vi "Aiming v2.vi"(6 "PID Cluster":T2={"L1 to L4 PID Cluster"={"L1 PID Gains"={"Kp"=0.005, "Kd"=0.5, "Ki"=0.0005}, "L2 PID Gains"={"Kp"=0.01, "Kd"=1.0, "Ki"=0.005}, "L3 PID Gains"={"Kp"=0.05, "Kd"=1.0, "Ki"=0.0005}, "L4 PID Gains"={"Kp"=0.1, "Kd"=0.1, "Ki"=0.0005}}, "Stage PID Cluster"={"Stage Z PID"={"Kp"=0.0005, "Kd"=0.001, "Ki"=0.0}, "Stage Y PID"={"Kp"=0.0003, "Kd"=0.01, "Ki"=0.0}, "Stage X PID"={"Kp"=0.0003, "Kd"=0.01, "Ki"=0.0}}, "OCT Z PID Gains"={"Kp"=0.0003, "Kd"=0.0001, "Ki"=0.01}}, 7 "Robot In":i32, 8 "error in":errorcluster, 9 "Aiming Pt":dbl[](array[numeric])=[0.0, 0.0, 0.0, 0.0], 10 "Prev Posit Cluster":T3={"Prev L1 to L4 Posit"=[0.0, 0.0, 0.0, 0.0], "Prev Stage Posit"=[6.0, 6.0, 6.0], "Prev OCT Z Posit"=0.0}, 11 "FPGA VI Reference In":refnum<k20>) -> (0 "error out":errorcluster, 2 "Last Posit Cluster":T1={"Last L1 to L4 Posit"=[0.0, 0.0, 0.0, 0.0], "Last Stage Posit"=[6.0, 6.0, 6.0], "Last OCT Z Posit"=0.0}, 3 "FPGA VI Reference Out":refnum<k20>)   [LabVIEW 2016]
uses:
  Subsystems/Global Variables.vi
  <vilib>/Platform/TimedLoop/XDataNode/wakeup.ctl
  <vilib>/Platform/TimedLoop/XDataNode/XDNodeRunTimeDep.lvlib
  <vilib>/Platform/TimedLoop/XDataNode/nitl_modes.ctl
  <vilib>/Platform/TimedLoop/XDataNode/timing_clust.ctl
  <vilib>/platform/TimedLoop/XDataNode/XDataNode.xnode
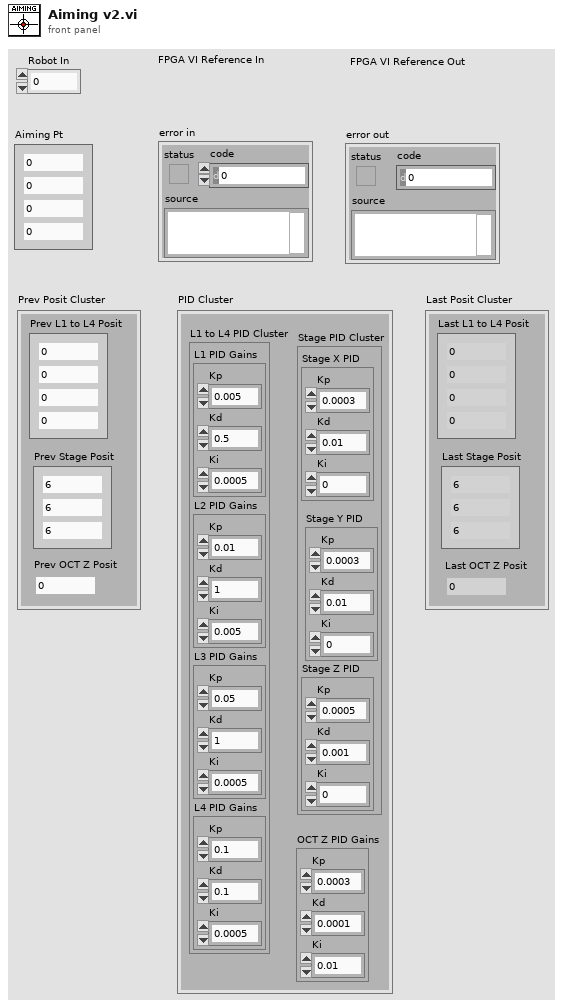
[diagram p1: front panel]
types:
  T1 = cluster{"Last L1 to L4 Posit":dbl[], "Last Stage Posit":dbl[], "Last OCT Z Posit":dbl}
  T2 = cluster{"L1 to L4 PID Cluster":cluster{"L1 PID Gains":cluster{"Kp":dbl, "Kd":dbl, "Ki":dbl}, "L2 PID Gains":cluster{"Kp":dbl, "Kd":dbl, "Ki":dbl}, "L3 PID Gains":cluster{"Kp":dbl, "Kd":dbl, "Ki":dbl}, "L4 PID Gains":cluster{"Kp":dbl, "Kd":dbl, "Ki":dbl}}, "Stage PID Cluster":cluster{"Stage Z PID":cluster{"Kp":dbl, "Kd":dbl, "Ki":dbl}, "Stage Y PID":cluster{"Kp":dbl, "Kd":dbl, "Ki":dbl}, "Stage X PID":cluster{"Kp":dbl, "Kd":dbl, "Ki":dbl}}, "OCT Z PID Gains":cluster{"Kp":dbl, "Kd":dbl, "Ki":dbl}}
  T3 = cluster{"Prev L1 to L4 Posit":dbl[], "Prev Stage Posit":dbl[], "Prev OCT Z Posit":dbl}
  T4 = typedef "XDNodeRunTimeDep.lvlib/timing_clust.ctl" = cluster{"Expected End [f-1]":u64, "Actual End [f-1]":u64, "Finished Late? [f-1]":bool, "Expected End [i-1]":u64, "Actual End [i-1]":u64, "Finished Late? [i-1]":bool, "Expected Start [i]":u64, "Actual Start [i]":u64, "Expected Start [f]":u64, "Actual Start [f]":u64, "Source Name":string, "Structure Name":string, "Period":i64, "Deadline":i64, "Offset":i64, "Start":i64, "Priority":i32, "Timeout":i32, "Mode":T5, "Wakeup Reason":T6, "Error":errorcluster, "Source Type":string, "Secondary Source Type":string, "Global End Time":u64, "Global Start Time":u64, "Frame Duration":u64, "Iteration Duration":u64, "Assigned CPU":i32, "I/O Scan Engine Mode":u32}
  T5 = typedef "XDNodeRunTimeDep.lvlib/nitl_modes.ctl" = enum32{"No Change", "Process missed periods, maintain original phase", "Discard missed periods, maintain original phase", "Process missed periods, ignore original phase", "Discard missed periods, ignore original phase"}
  T6 = typedef "XDNodeRunTimeDep.lvlib/wakeup.ctl" = enum32{"Normal", "Aborted", "Asynchronous wakeup", "Timing source error", "Timed loop error", "Timeout"}
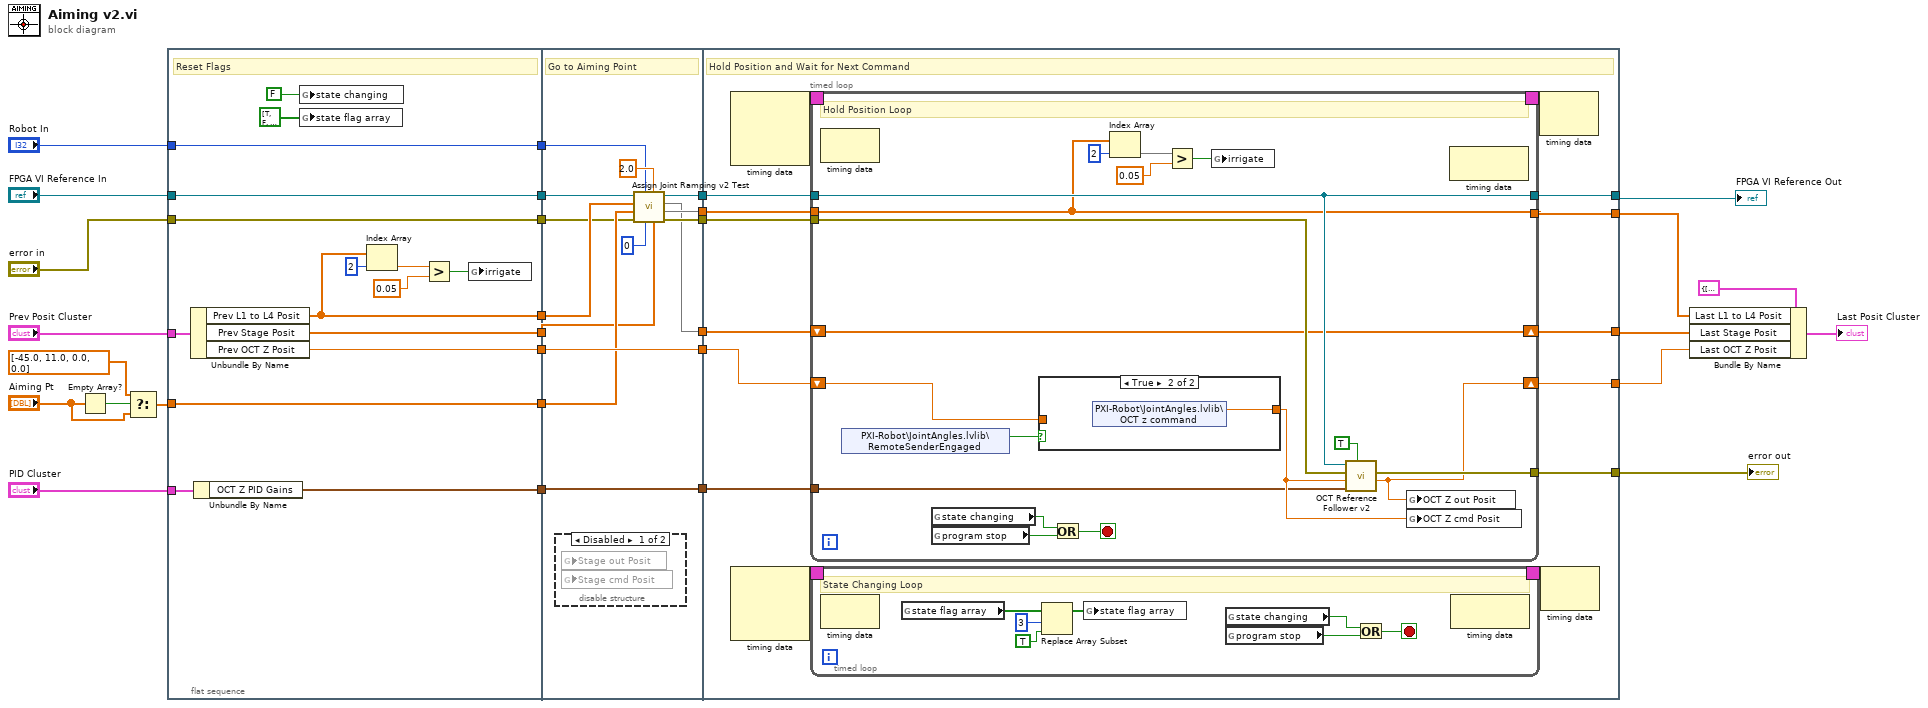
[diagram p0: block diagram]
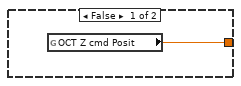
[diagram p3: hidden frame]
diagram:
  n1 = Empty Array?(array="Aiming Pt") -> (empty?=w24:bool)
  n2 = Select(t=dbl[] [-45.0, 11.0, 0.0, 0.0] ("First Trk Pt 2"), s=w24, f="Aiming Pt") -> (s? t:f=w21:dbl[])
  n3 = flat-sequence {
    tunnel: [w44] -> w30
    tunnel: "FPGA VI Reference In" -> [w44]
    tunnel: "error in" -> [w43]
    tunnel: [w43] -> w29
    tunnel: [w31] -> w28
    tunnel: "PID Cluster" -> [w38]
    tunnel: [w39] -> w26
    tunnel: w21 -> [w39]
    tunnel: "Prev Posit Cluster" -> [w42]
    tunnel: [w41] -> w9
    tunnel: [w40] -> w6
    tunnel: [w37] -> w5
    tunnel: "Robot In" -> [w36]
    tunnel: [w36] -> w1
    tunnel: w30 -> [w55]
    tunnel: w29 -> [w52]
    tunnel: w28 -> [w54]
    tunnel: w26 -> [w53]
    tunnel: [w56] -> w25
    tunnel: [w58] -> w20
    tunnel: [w59] -> w17
    tunnel: w9 -> [w48]
    tunnel: [w47] -> w8
    tunnel: [w60] -> w7
    tunnel: w6 -> [w60]
    tunnel: w5 -> [w59]
    tunnel: [w57] -> w4
    tunnel: w1 -> [w50]
    tunnel: [w71] -> w13
    tunnel: w25 -> [w72]
    tunnel: w20 -> [w73]
    tunnel: [w63] -> w18
    tunnel: [w70] -> w19
    tunnel: w17 -> [w69]
    tunnel: [w68] -> w14
    tunnel: [w67] -> w3
    tunnel: w8 -> [w66]
    tunnel: w7 -> [w65]
    tunnel: w4 -> [w64]
    frame #0 {
      # "Reset Flags"
      n4 = Unbundle By Name(w42) -> ("Prev L1 to L4 Posit"=w31:dbl[], "Prev Stage Posit"=w41:dbl[], "Prev OCT Z Posit"=w40:dbl)
      n5 = Unbundle By Name(w38) -> ("OCT Z PID Gains"=w37:cluster{"Kp":dbl, "Kd":dbl, "Ki":dbl})
      n6 = global write "Global Variables.vi" "state changing"(FALSE ("state changing")) -> ()
      n7 = global write "Global Variables.vi" "state flag array"(bool[] [TRUE, FALSE, FALSE, FALSE, FALSE, FALSE, FALSE, FALSE, FALSE] ("state flag array")) -> ()
      n8 = Index Array(array=w31, index=2) -> (element=w34:dbl)
      n9 = Greater?(x=w34, y=0.05) -> (0:w33:bool)
      n10 = global write "Global Variables.vi" "irrigate"(w33) -> ()
    }
    frame #1 {
      # "Go to Aiming Point"
      n11 = disable-structure shown="Disabled" {
        frame Disabled {
          n12 = global read "Global Variables.vi" "Stage out Posit"() -> ()  [unwired: 1 in]
          n13 = global read "Global Variables.vi" "Stage cmd Posit"() -> ()  [unwired: 1 in]
        }
        frame Enabled {
        }
      }
      n14 = call "Assign Joint Ramping v2 Test.vi"(4:w48, "Ramp Time [sec]"=2.0, "Vac Digital Cmd"=i8 0, "Robot In"=w50, "error in"=w52, "Destination Posit Array [mm]"=w53, 10:w54, "FPGA VI Reference In"=w55) -> ("error out"=w56:errorcluster, 1:w57, 2:w47, "FPGA VI Reference Out"=w58:refnum<k20>)
    }
    frame #2 {
      # "Hold Position and Wait for Next Command"
      n15 = node-c288() -> (w75:T4)  [unwired: 3 in]
      n16 = node-c288() -> (w62:T4)  [unwired: 3 in]
      n17 = timed-loop {
        timing: w75 -> [_]
        timing-out: [_] -> w74
        tunnel: w73 -> [w96]
        tunnel: w72 -> [w95]
        tunnel: [w96] -> w71
        tunnel: w69 -> [w99]
        tunnel: [w98] -> w67
        shift-right: [w87] -> w70
        shift-left: w66 -> [w87]
        shift-right: [w97] -> w68
        shift-left: w65 -> [w101]
        tunnel: w64 -> [w88]
        tunnel: [w88] -> w63
        stop <- w102 stop-if-true
        # "Hold Position Loop"
        n18 = node-c288() -> ()  [unwired: 1 in, 1 out]
        n19 = shared-variable "PXI-Robot\\JointAngles.lvlib\\RemoteSenderEngaged"() -> (w94:bool)  [unwired: 1 in, 1 out]
        n20 = global read "Global Variables.vi" "state changing"() -> (w104:bool)
        n21 = global read "Global Variables.vi" "program stop"() -> (w103:bool)
        n22 = case shown="True" w94 {
          tunnel: [w105 w106] -> w100
          tunnel: w101 -> [_ _]
          frame False {
            # "Hold Position if not Engaged"
            n23 = global read "Global Variables.vi" "OCT Z cmd Posit"() -> (w105:dbl)
          }
          frame True {
            n24 = shared-variable "PXI-Robot\\JointAngles.lvlib\\OCT z command"() -> (w106:dbl)  [unwired: 1 in, 1 out]
          }
        }
        n25 = Or(x=w104, y=w103) -> (x .or. y?=w102:bool)
        n26 = Index Array(array=w88, index=2) -> (element=w91)
        n27 = Greater?(x=w91, y=0.05) -> (0:w90:bool)
        n28 = global write "Global Variables.vi" "irrigate"(w90) -> ()
        n29 = call "OCT Reference Follower v2.vi"("OCT Act ON"=TRUE, "OCT Z PID Gains"=w99, "OCT  Z cmd Posit [mm]"=w100, "error in"=w95, "FPGA VI Reference In"=w96) -> ("OCT  Z out Posit [mm]"=w97:dbl, "error out"=w98:errorcluster)  [unwired: 4 in, 1 out]
        n30 = global write "Global Variables.vi" "OCT Z out Posit"(w97) -> ()
        n31 = global write "Global Variables.vi" "OCT Z cmd Posit"(w100) -> ()
        n32 = node-c288() -> ()  [unwired: 1 in, 1 out]
      }
      n33 = timed-loop {
        timing: w62 -> [_]
        timing-out: [_] -> w61
        stop <- w76 stop-if-true
        # "State Changing Loop"
        n34 = node-c288() -> ()  [unwired: 1 in, 1 out]
        n35 = global read "Global Variables.vi" "state flag array"() -> (w81:bool[])
        n36 = Replace Array Subset(array=w81, new element=TRUE ("new element/subarray"), index=3) -> (w80:bool[])
        n37 = global write "Global Variables.vi" "state flag array"(w80) -> ()
        n38 = global read "Global Variables.vi" "state changing"() -> (w82:bool)
        n39 = global read "Global Variables.vi" "program stop"() -> (w77:bool)
        n40 = Or(x=w82, y=w77) -> (x .or. y?=w76:bool)
        n41 = node-c288() -> ()  [unwired: 1 in, 1 out]
      }
      n42 = node-c288(w74) -> ()  [unwired: 1 out]
      n43 = node-c288(w61) -> ()  [unwired: 1 out]
    }
  }
  n44 = Bundle By Name(cluster=T1 {"Last L1 to L4 Posit"=[0.0, 0.0, 0.0, 0.0], "Last Stage Posit"=[6.0, 6.0, 6.0], "Last OCT Z Posit"=0.0} ("Last Posit Cluster 2"), "Last L1 to L4 Posit"=w18, "Last Stage Posit"=w19, "Last OCT Z Posit"=w14) -> (→"Last Posit Cluster":T1)
  "FPGA VI Reference Out" <- w13
  "error out" <- w3
